vi "Handle Add State Change.vi"(8 "error in (no error)":errorcluster, 9 "Duplicate State":bool, 10 "State":string, 11 "Routing Channel Ref in":T1 format="%.0x") -> (0 "error out":errorcluster, 1 "New State Added":string, 3 "Routing Channel Ref out":T1 format="%.0x")   [LabVIEW 2017, in "Routing and Faulting System Explorer.lvlib"]
uses:
  Routing and Faulting System Explorer.lvlib
  Scripting/Routing and Faulting Scripting.lvlib
  Shared/Connection.ctl
  Shared/Routing and Faulting Shared.lvlib
  Shared/Routing State.ctl
  <vilib>/NI Veristand/Custom Device API/Custom Device Item Ref.ctl
  <vilib>/NI VeriStand/Custom Device API/Custom Device API.lvlib
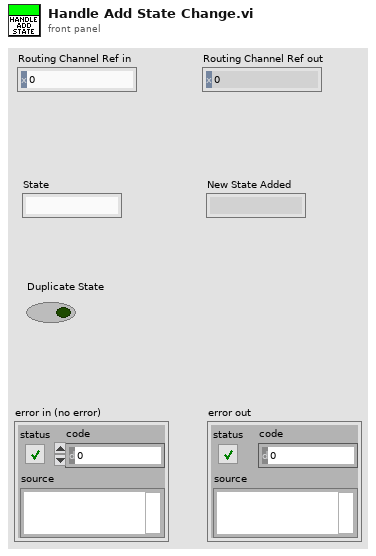
[diagram p1: front panel]
types:
  T1 = typedef "Custom Device API.lvlib/Custom Device Item Ref.ctl" = u64
  T2 = typedef "Routing and Faulting Shared.lvlib/Routing State.ctl" = cluster{"Name":string, "Description":string, "Value":i32, "Connection List":T3[]}
  T3 = typedef "Routing and Faulting Shared.lvlib/Connection.ctl" = cluster{"Resource":string, "Source":string, "Destination":string}
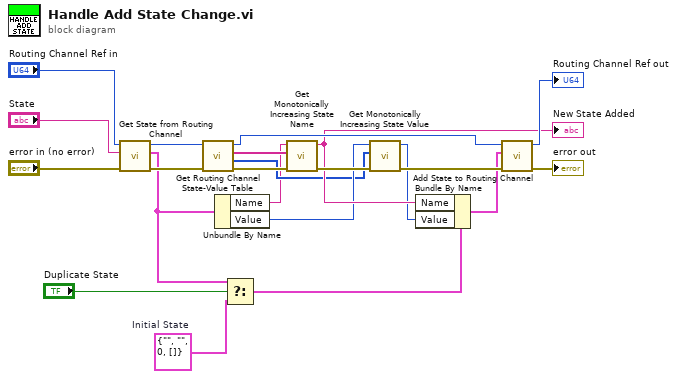
[diagram p0: block diagram]
diagram:
  w1 = T2 {"Name"="", "Description"="", "Value"=0, "Connection List"=[]}  # Initial State
  n1 = call "Get State from Routing Channel.vi"("error in (no error)"="error in (no error)", "State"="State", "Channel Ref in"="Routing Channel Ref in") -> ("error out"=w18:errorcluster, "State and Connections"=w3:T2, "Channel Ref out"=w19:T1)  [unwired: 6 in]
  n2 = call "Get Routing Channel State-Value Table.vi"("error in (no error)"=w18, "Channel Ref in"=w19) -> ("error out"=w17:errorcluster, "State Values"=w7:i32[], "State Names"=w6:string[], "Channel Ref out"=w14:T1)  [unwired: 6 in]
  n3 = Unbundle By Name(w3) -> ("Name"=w5:string, "Value"=w8:i32)
  n4 = Select(t=w3, s="Duplicate State", f=w1) -> (s? t:f=w2:T2)
  n5 = call "Get Monotonically Increasing State Name.vi"("error in (no error)"=w17, "State Names"=w6, "Desired State Name"=w5) -> ("error out"=w20:errorcluster, "New State Name"=w10:string)  [unwired: 7 in]
  "New State Added" <- w10
  n6 = call "Get Monotonically Increasing State Value.vi"("error in (no error)"=w20, "State Values"=w7, "Desire State Value"=w8) -> ("error out"=w16:errorcluster, "New State Value"=w9:i32)  [unwired: 7 in]
  n7 = Bundle By Name(cluster=w2, "Name"=w10, "Value"=w9) -> (w12:T2)
  n8 = call "Add State to Routing Channel.vi"("error in (no error)"=w16, "State and Connections"=w12, "Channel Ref in"=w14) -> ("error out"=→"error out":errorcluster, "Channel Ref out"=→"Routing Channel Ref out":T1)  [unwired: 7 in]
